vi "New BuildWorker.vi"(7 "BuildWorker in":refnum<class "BuildWorker.lvclass">, 8 "error in (no error)":errorcluster, 10 "BuildServer Port":u16, 11 "Name":string) -> (0 "error out":errorcluster, 3 "BuildWorker out":refnum<class "BuildWorker.lvclass">)   [LabVIEW 2017, in "BuildWorker.lvlib" / "BuildWorker.lvclass"]
uses:
  BuildWorker.lvclass
  BuildWorker.lvclass/BuildWorker.ctl
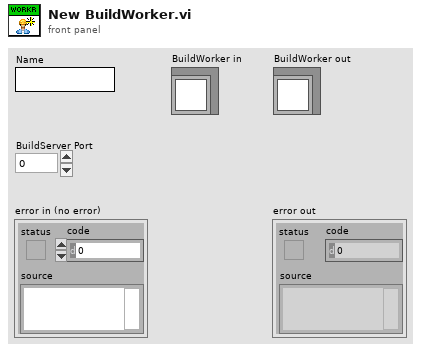
[diagram p1: front panel]
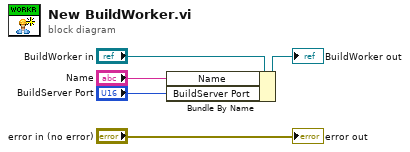
[diagram p0: block diagram]
diagram:
  n1 = Bundle By Name(cluster="BuildWorker in", "Name"="Name", "BuildServer Port"="BuildServer Port") -> (→"BuildWorker out":refnum<class "BuildWorker.lvclass">)
  "error out" <- "error in (no error)"
